vi "Read Roles.vi"(8 "error in (no error)":errorcluster, 11 "5RobotsNormalGamePlay in":refnum<class "5RobotsNormalGamePlay.lvclass">) -> (0 "error out":errorcluster, 2 "Roles":T1, 3 "5RobotsNormalGamePlay out":refnum<class "5RobotsNormalGamePlay.lvclass">)   [LabVIEW 2020, in "5RobotsNormalGamePlay.lvclass"]
uses:
  5RobotsNormalGamePlay.lvclass
  ShootRole_class/ShootRole.lvclass
  FollowAttackerRole_class/FollowAttackerRole.lvclass
  PassObserverRole_class/PassObserverRole.lvclass
  PreparePassReceiverRole_class/PreparePassReceiverRole.lvclass
  5RobotsNormalGamePlay.lvclass/5RobotsNormalGamePlay.ctl
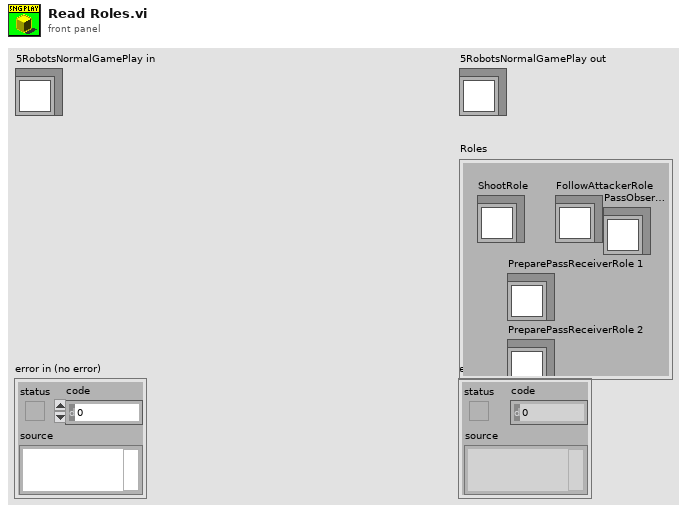
[diagram p1: front panel]
types:
  T1 = cluster{"ShootRole":refnum<class "ShootRole.lvclass">, "FollowAttackerRole":refnum<class "FollowAttackerRole.lvclass">, "PassObserverRole":refnum<class "PassObserverRole.lvclass">, "PreparePassReceiverRole 1":refnum<class "PreparePassReceiverRole.lvclass">, "PreparePassReceiverRole 2":refnum<class "PreparePassReceiverRole.lvclass">}
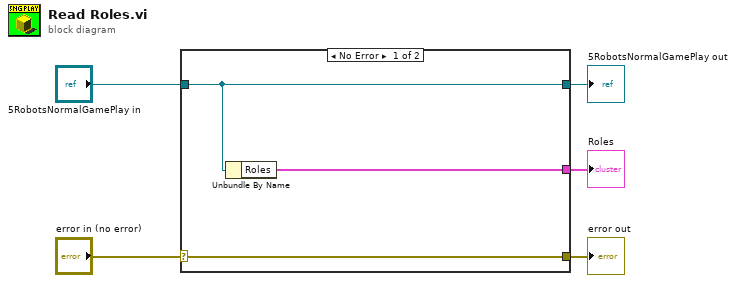
[diagram p0: block diagram]
diagram:
  n1 = case shown="No Error" "error in (no error)" {
    selector: "error in (no error)" -> [w8 w9]
    tunnel: [w8 w9] -> w4
    tunnel: [w7 w10] -> w2
    tunnel: "5RobotsNormalGamePlay in" -> [w7 w10]
    tunnel: [w6 _] -> w1
    frame No Error {
      n2 = Unbundle By Name(w7) -> ("Roles"=w6:T1)
    }
    frame Error {
    }
  }
  "error out" <- w4
  "5RobotsNormalGamePlay out" <- w2
  "Roles" <- w1
